vi "输出调用02.vi"(0 "输出簇":cluster{"用户名":string, "项目名称":string}, 7 "数组":string[][](array[string]), 9 "字符串":string, 11 "输出簇 2":T1, 12 "Str引用句柄":refnum<vi>) -> ()   [LabVIEW 2020]
uses:
  <vilib>/Utility/miscctls.llb/LVDateTimeRec.ctl
  <vilib>/numeric/Random Number (Range) DBL.vi
panel:
  out "压力":dbl
  out "数组 6":dbl[][](array[numeric])
  out "水质":dbl
  out "温度":dbl
  out "输出 3":dbl
  out "输出 2":dbl
  out "创建的路径":path
  out "路径 2":path
  out "路径":path
  out "错误输出":errorcluster
  out "数组 5":dbl[](array[numeric])
  out "数组 4":dbl[](array[numeric])
  out "文本":string[](array[string])
  out "数组 3":dbl[](array[numeric])
  out "数组 2":dbl[](array[numeric])
  out "错误输出 2":errorcluster caption="错误输出"
  out "元素":string
  out "数值 3":i32
  out "Numeric":i32
  in  "数值":u32
  out "输出 1":dbl
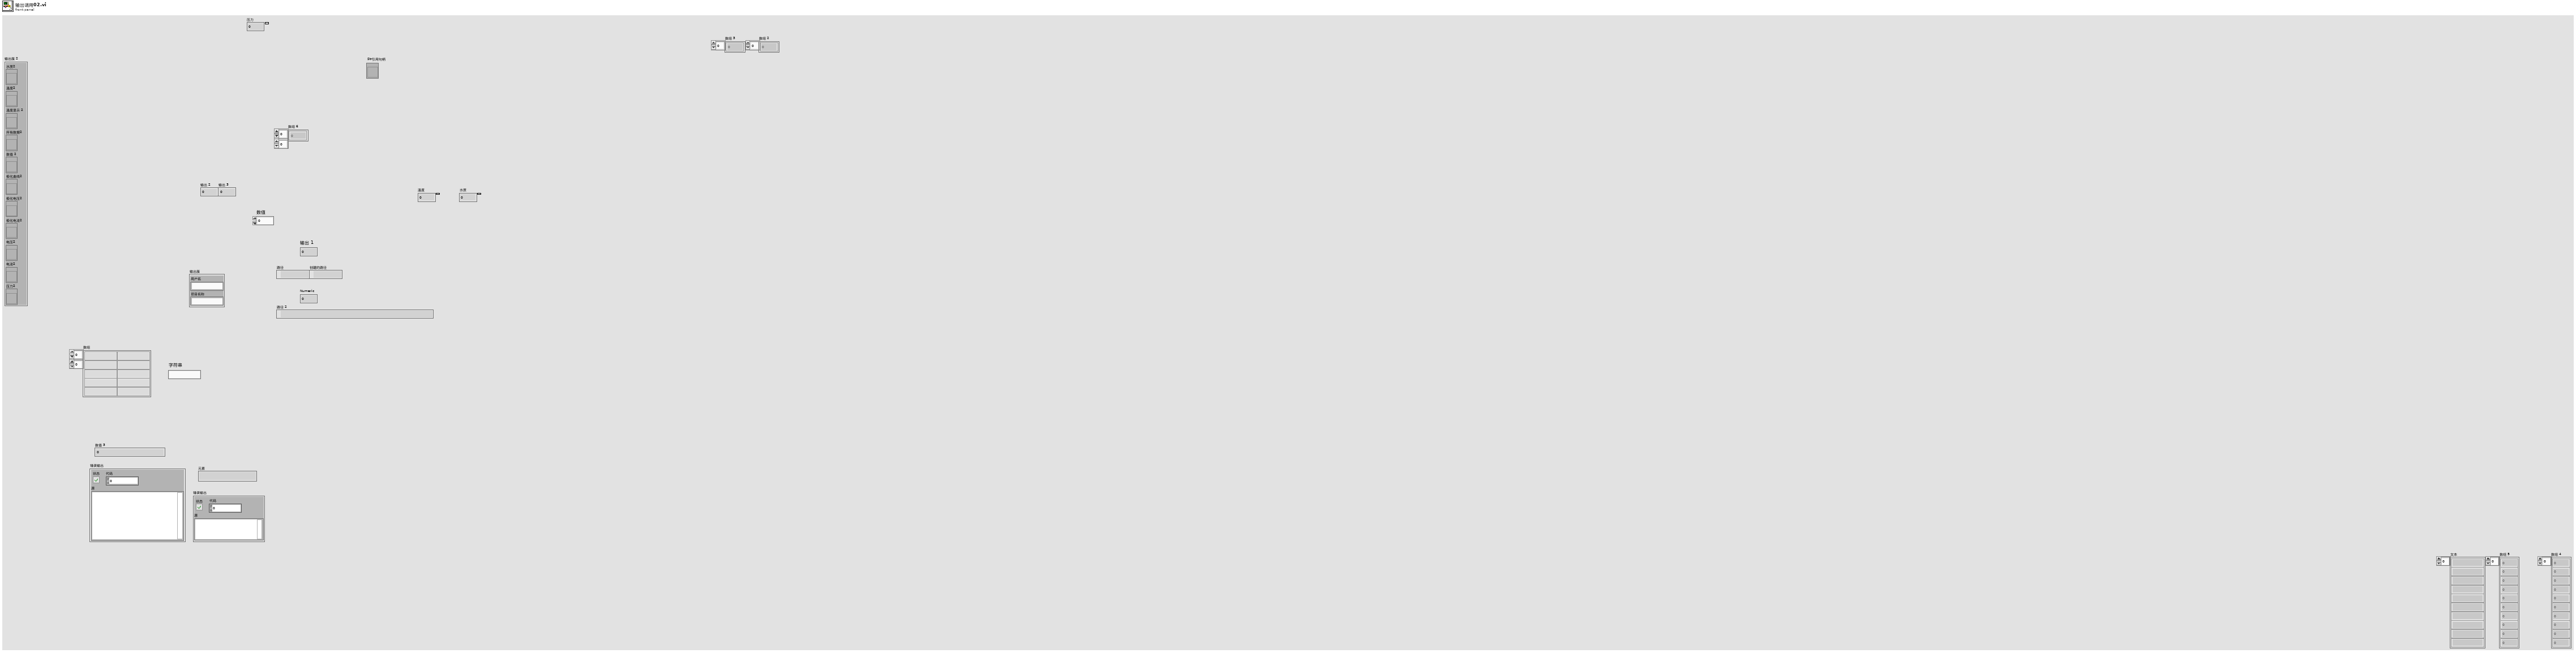
[diagram p1: front panel]
types:
  T1 = cluster{"水质2":refnum<vi>, "温度2":refnum<vi>, "温度显示 2":refnum<vi>, "所有数据2":refnum<vi>, "数值 2":refnum<vi>, "极化曲线2":refnum<vi>, "极化电压2":refnum<vi>, "极化电流2":refnum<vi>, "电压2":refnum<vi>, "电流2":refnum<vi>, "压力2":refnum<vi>}
  T2 = enum16{"open", "replace", "create", "open or create", "replace or create", "replace or create with confirmation"}
  T3 = typedef "LVDateTimeRec.ctl" = cluster{"fractional second":dbl, "second":i32, "minute":i32, "hour":i32, "day of month":i32, "month":i32, "year":i32, "day of week":i32, "day of year":i32, "DST":i32}
  T4 = enum16{"open", "open or create", "create or replace", "create", "open (read-only)"}
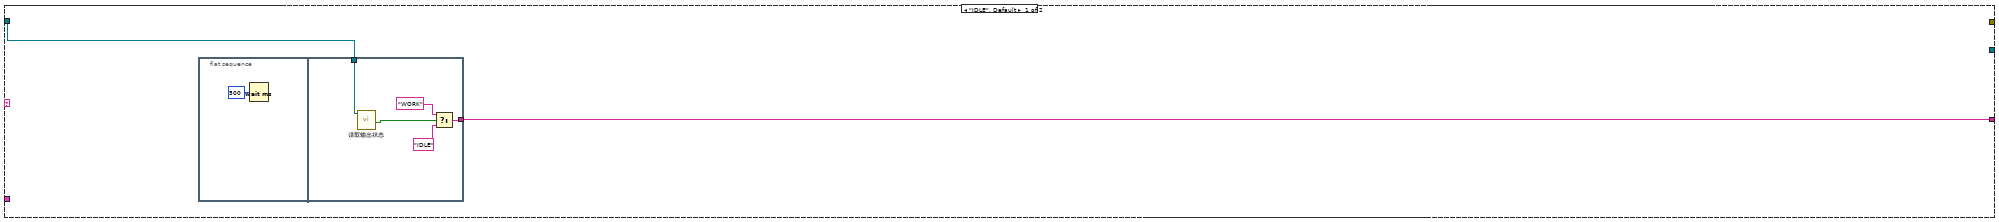
[diagram p2: hidden frame]
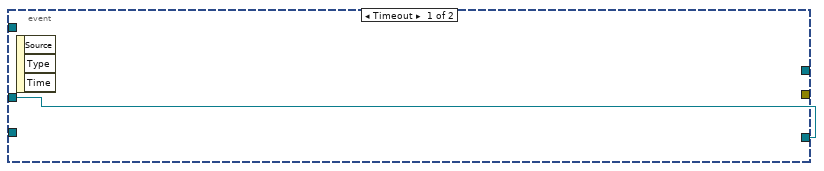
[diagram p3: hidden frame]
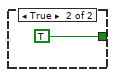
[diagram p5: hidden frame]
diagram:
  w17 = "\\" ("string")
  (unwired) dbl[] [] ("数组 4")
  n1 = Unbundle By Name("输出簇") -> ("用户名"=w14:string, "项目名称"=w13:string)
  n2 = Get Date/Time In Seconds() -> (seconds since 1Jan1904=w35:timestamp)
  n3 = Format Date/Time String(time format string (%c)="%y-%m-%d[%H-%M]", seconds (now)=w35) -> (date/time string=w16:string)  [unwired: 1 in]
  n4 = Concatenate Strings("C:\\Users\\526computer\\Desktop", w17, "TEMPDATA\\" ("string"), w14, w17, w13, w17, "CH2\\" ("string"), w16) -> (w33:string)
  n5 = String To Path(string=w33) -> (path=w32:path)
  n6 = Create Folder(path (use dialog)=w32) -> (created path=w4:path)  [unwired: 2 in, 2 out]
  "创建的路径" <- w4
  n7 = Path To String(path=w4) -> (string=w31:string)
  n8 = Concatenate Strings(w31, "\\" ("string"), "索引02.txt" ("string")) -> (w23:string)
  n9 = Path To String(path=w4) -> (string=w2:string)
  n10 = String To Path(string=w23) -> (path=w22:path)
  "路径 2" <- w22
  n11 = property on="输出簇 2" class="Clust (严格)"() -> ("Value"=w6:T1)  [unwired: 2 in, 2 out]
  n12 = property class="Str"(reference="Str引用句柄", "Value"=w2) -> ()  [unwired: 1 in, 2 out]
  n13 = Unbundle By Name(w6) -> ("极化曲线2"=w12:refnum<vi>)
  n14 = property on="数组 6" class="Arr (严格)"("Value"=dbl[][] [] ("数组 6")) -> (error out=w8:errorcluster)  [unwired: 2 in, 1 out]
  n15 = Open/Create/Replace File(file path (use dialog)=w22, operation (0:open)=T2."replace or create") -> (refnum out=w21:refnum<file>)  [unwired: 4 in, 2 out]
  n16 = while {
    tunnel: w45 -> [w66]
    tunnel: w21 -> [w65]
    tunnel: [w64] -> w19
    tunnel: [w63] -> w20
    shift-right: [w61] -> _
    shift-left: w12 -> [w62]
    tunnel: w8 -> [_]
    stop <- FALSE stop-if-true
    n17 = event shown="[1] \"数值\": 值改变" {
      selector: _ -> [_ _]
      dyn-events: _ -> [_ _]
      timeout: 100 -> [_ _]
      tunnel: w66 -> [_ _]
      tunnel: w65 -> [_ w84]
      tunnel: [_ w78] -> w64
      tunnel: [_ w77] -> w63
      tunnel: w62 -> [w69 w73]
      tunnel: [w69 w72] -> w61
      event Timeout {
        n18 = event-data() -> ()  [unwired: 1 in, 3 out]
      }
      event "数值": Value Change {
        n19 = event-data() -> ()  [unwired: 1 in, 6 out]
        n20 = local read "输出 3"() -> (w74:dbl)
        n21 = local read "输出 2"() -> (w75:dbl)
        n22 = property on="Numeric" class="DigNum (严格)"() -> ("Value"=w83:i32)  [unwired: 2 in, 2 out]
        n23 = Build Array(w75, w74) -> (w76:dbl[])
        n24 = Format Into String(w83) -> (resulting string=w82:string)  [unwired: 3 in, 1 out]
        n25 = property on="数组 6" class="Arr (严格)"() -> ("Value"=w71:dbl[][])  [unwired: 2 in, 2 out]
        n26 = Write to Text File(file (use dialog)=w84, text=w82) -> (refnum out=w81:refnum<file>, error out=w80:errorcluster)  [unwired: 2 in, 1 out]
        n27 = Insert Into Array(array=w71, new element=w76) -> (w70:dbl[][])  [unwired: 2 in]
        n28 = property on="数组 6" class="Arr (严格)"("Value"=w70) -> ()  [unwired: 2 in, 2 out]
        n29 = Write to Text File(file (use dialog)=w81, text="\r\n", error in=w80) -> (refnum out=w78:refnum<file>, error out=w77:errorcluster)  [unwired: 1 in, 1 out]
        n30 = property class="Arr (严格)"(reference=w73, "Value"=w70) -> (reference out=w72:refnum<vi>)  [unwired: 1 in, 1 out]
      }
    }
  }
  n31 = Path To String(path=w4) -> (string=w26:string)
  n32 = Concatenate Strings(w26, "\\" ("string"), "数据02.txt" ("string")) -> (w25:string)
  n33 = String To Path(string=w25) -> (path=w24:path)
  "路径" <- w24
  n34 = Close File(refnum=w19, error in=w20) -> ()  [unwired: 2 out]
  n35 = Open/Create/Replace File(file path (use dialog)=w24, operation (0:open)=T2."replace or create" ("操作(0:open)")) -> (refnum out=w10:refnum<file>, error out=w40:errorcluster)  [unwired: 4 in, 1 out]
  n36 = flat-sequence {
    tunnel: [w89] -> w60
    tunnel: [w86] -> w57
    tunnel: w60 -> [w93]
    tunnel: [w93] -> w59
    tunnel: [w92] -> w58
    tunnel: w57 -> [w92]
    tunnel: ["字符串"] -> w43
    tunnel: w59 -> [w95]
    tunnel: w58 -> [w96]
    tunnel: [w96] -> w56
    tunnel: [w95] -> w55
    tunnel: [w94] -> w44
    tunnel: w43 -> [w94]
    tunnel: w56 -> [w103]
    tunnel: w55 -> [w104]
    tunnel: [w106] -> w54
    tunnel: [w105] -> w53
    tunnel: [w104] -> w51
    tunnel: [w103] -> w49
    tunnel: [w102] -> w45
    tunnel: w44 -> [w101]
    tunnel: w54 -> [w119]
    tunnel: w53 -> [w118]
    tunnel: [w115] -> w52
    tunnel: w51 -> [w115]
    tunnel: [w114] -> w50
    tunnel: w49 -> [w114]
    tunnel: [w109] -> w48
    tunnel: [w108] -> w47
    tunnel: ["输出簇 2"] -> w11
    tunnel: w52 -> [w148]
    tunnel: w50 -> [w152]
    tunnel: w48 -> [w151]
    tunnel: w47 -> [w150]
    tunnel: [w149] -> w46
    tunnel: [w145] -> w37
    tunnel: w11 -> [w144]
    tunnel: w46 -> [w205]
    tunnel: w37 -> [w203]
    frame #0 {
      n37 = property on="数值" class="DigNum (严格)"("Value"=i64 0 ("数值")) -> ()  [unwired: 2 in, 2 out]
      n38 = Index Array(array="数组", index (col)=5 ("禁用的索引 (列)")) -> (element=w86:string[])  [unwired: 1 in]
      n39 = Index Array(array="数组", index (col)=3 ("禁用的索引 (列)")) -> (element=w89:string[])  [unwired: 1 in]
    }
    frame #1 {
      n40 = VISA Close(VISA resource name="字符串") -> ()  [unwired: 1 in, 1 out]
    }
    frame #2 {
    }
    frame #3 {
      n41 = VISA Open(VISA resource name=w101) -> (VISA resource name=w102:refnum<visa-resource-name>, error out=w99:errorcluster)  [unwired: 4 in]
      n42 = call "remote.vi"("error in (no error)"=w99, "VISA resource name"=w102) -> ("error out"=w97:errorcluster, "VISA resource name out"=w98:refnum<visa-resource-name>)  [unwired: 8 in]
      n43 = call "enableoutput.vi"("error in (no error)"=w97, "Enable OutPut(True)"=FALSE, "VISA resource name"=w98) -> ("error out"=w105:errorcluster, "VISA resource name out"=w106:refnum<visa-resource-name>)  [unwired: 7 in]
    }
    frame #4 {
      n44 = flat-sequence {
        tunnel: w119 -> [w124]
        tunnel: w118 -> [w123]
        tunnel: [w121] -> w117
        tunnel: [w120] -> w116
        tunnel: w117 -> [w130]
        tunnel: w116 -> [w129]
        tunnel: [w126] -> w113
        tunnel: [w125] -> w112
        tunnel: w113 -> [w136]
        tunnel: w112 -> [w135]
        tunnel: [w133] -> w111
        tunnel: [w132] -> w110
        tunnel: w111 -> [w142]
        tunnel: w110 -> [w141]
        tunnel: [w138] -> w109
        tunnel: [w137] -> w108
        frame #0 {
          n45 = call "priority.vi"("error in (no error)"=w123, "字符串"="CURR", "VISA resource name"=w124) -> ("error out"=w120:errorcluster, "VISA resource name out"=w121:refnum<visa-resource-name>)  [unwired: 7 in]
        }
        frame #1 {
          n46 = call "初始化电压电流.vi"("error in (no error)"=w129, "输入 2"=0.1, "输入 1"=15.0, "VISA resource name"=w130) -> ("error out"=w125:errorcluster, "VISA resource name out"=w126:refnum<visa-resource-name>)  [unwired: 6 in]
        }
        frame #2 {
          n47 = call "限制电流.vi"("error in (no error)"=w135, "OCP Delay(0)"=3.0, "数值"=120.0 ("OCP Level(0)"), "VISA resource name"=w136) -> ("error out"=w132:errorcluster, "VISA resource name out"=w133:refnum<visa-resource-name>)  [unwired: 6 in]
        }
        frame #3 {
          n48 = call "限制电压.vi"("error in (no error)"=w141, "OVP Delay(0)"=3.0, "OVP Level(0)"=20.0, "VISA resource name"=w142) -> ("error out"=w137:errorcluster, "VISA resource name out"=w138:refnum<visa-resource-name>)  [unwired: 6 in]
        }
      }
    }
    frame #5 {
      n49 = Unbundle By Name(w144) -> ("数值 2"=w143:refnum<vi>)
      n50 = Search 1D Array(1D array=w148, element=" " ("元素")) -> (index of element=w146:i32)  [unwired: 1 in]
      n51 = for {
        N: w146 -> [_]
        tunnel: w152 -> [w174] mode=indexing
        tunnel: w148 -> [w171] mode=indexing
        tunnel: w150 -> [w169]
        shift-right: [w164] -> w149
        shift-left: w151 -> [w170]
        tunnel: [w161] -> w145
        shift-right: [w155] -> _
        shift-left: w143 -> [w156]
        i -> [w154]
        n52 = Scan From String(input string=w174) -> (output 1=w173:dbl)  [unwired: 4 in, 3 out]
        n53 = Scan From String(input string=w171) -> (output 1=w168:dbl)  [unwired: 4 in, 3 out]
        "输出 1" <- w168
        n54 = Multiply(x=w173, y=1000.0) -> (x*y=w165:dbl)
        n55 = flat-sequence {
          tunnel: w170 -> [w179]
          tunnel: w169 -> [w178]
          tunnel: w168 -> [w177]
          tunnel: [w176] -> w167
          tunnel: [w175] -> w166
          tunnel: w167 -> [w182]
          tunnel: w166 -> [w183]
          tunnel: [w181] -> w163
          tunnel: [w180] -> w162
          tunnel: w165 -> [w193]
          tunnel: w163 -> [w192]
          tunnel: [w192] -> w160
          tunnel: [w191] -> w158
          tunnel: w162 -> [w191]
          tunnel: w160 -> [w198]
          tunnel: [w198] -> w159
          tunnel: w158 -> [w197]
          tunnel: [w197] -> w157
          tunnel: w156 -> [w196]
          tunnel: [w195] -> w155
          tunnel: w153 -> [w194]
          tunnel: [w201] -> w164
          tunnel: w159 -> [w202]
          tunnel: w157 -> [w200]
          tunnel: [w199] -> w161
          frame #0 {
            n56 = call "设置电流.vi"("error in (no error)"=w178, "输入 1"=w177, "VISA resource name"=w179) -> ("error out"=w175:errorcluster, "VISA resource name out"=w176:refnum<visa-resource-name>)  [unwired: 7 in]
          }
          frame #1 {
            n57 = First Call?() -> (First Call?: T/F=w184:bool)
            n58 = case shown="真" w184 {
              tunnel: w182 -> [w185 w190]
              tunnel: w183 -> [_ w189]
              tunnel: [w185 w187] -> w181
              tunnel: [_ w186] -> w180
              frame False {
              }
              frame True {
                n59 = call "enableoutput.vi"("error in (no error)"=w189, "Enable OutPut(True)"=TRUE, "VISA resource name"=w190) -> ("error out"=w186:errorcluster, "VISA resource name out"=w187:refnum<visa-resource-name>)  [unwired: 7 in]
              }
            }
          }
          frame #2 {
            n60 = Wait (ms)(milliseconds to wait=w193) -> ()  [unwired: 1 out]
          }
          frame #3 {
            n61 = property on="数值" class="DigNum (严格)"("Val(Sgnl)"=w194) -> ()  [unwired: 2 in, 2 out]
            n62 = property class="DigNum (严格)"(reference=w196, "Val(Sgnl)"=w194) -> (reference out=w195:refnum<vi>)  [unwired: 1 in, 1 out]
          }
          frame #4 {
            n63 = call "remote.vi"("error in (no error)"=w200, "VISA resource name"=w202) -> ("error out"=w199:errorcluster, "VISA resource name out"=w201:refnum<visa-resource-name>)  [unwired: 8 in]
          }
        }
        n64 = Increment(x=w154) -> (x+1=w153:i32)
      }
    }
    frame #6 {
      n65 = flat-sequence {
        tunnel: w205 -> [w209]
        tunnel: [w208] -> w204
        tunnel: w203 -> [w206]
        tunnel: w204 -> [w210]
        frame #0 {
          n66 = call "enableoutput.vi"("error in (no error)"=w206, "Enable OutPut(True)"=FALSE, "VISA resource name"=w209) -> ("VISA resource name out"=w208:refnum<visa-resource-name>)  [unwired: 7 in, 1 out]
        }
        frame #1 {
          n67 = VISA Close(VISA resource name=w210) -> ()  [unwired: 1 in, 1 out]
        }
        frame #2 {
          n68 = flat-sequence {
            tunnel: [w227] -> w221
            tunnel: [w226] -> w220
            tunnel: [w225] -> w219
            tunnel: [w224] -> w218
            tunnel: [w223] -> w217
            tunnel: w221 -> [w270]
            tunnel: w220 -> [w269]
            tunnel: [w287] -> w211
            tunnel: [w286] -> w212
            tunnel: w219 -> [w282]
            tunnel: [w281] -> w213
            tunnel: w218 -> [w273]
            tunnel: w217 -> [w274]
            tunnel: [w271] -> w214
            tunnel: [w272] -> w215
            tunnel: [w271] -> w216
            tunnel: w216 -> [w328]
            tunnel: w215 -> [w327]
            tunnel: w214 -> [w349]
            tunnel: w213 -> [w355]
            tunnel: w212 -> [w363]
            tunnel: w211 -> [w362]
            frame #0 {
              n69 = property on="路径" class="Path"() -> ("Value"=w222:path)  [unwired: 2 in, 2 out]
              n70 = Open/Create/Replace File(file path (use dialog)=w222, operation (0:open)=T2."open" ("操作(0:open)")) -> (refnum out=w230:refnum<file>, error out=w229:errorcluster)  [unwired: 4 in, 1 out]
              n71 = while {
                tunnel: w230 -> [w266]
                tunnel: w229 -> [w264]
                tunnel: [w263] -> w228
                tunnel: [w237] -> w227 mode=indexing
                tunnel: [w236] -> w226 mode=indexing
                tunnel: [w252] -> _
                tunnel: [w240] -> w225 mode=indexing
                tunnel: [w235] -> w224 mode=indexing
                tunnel: [w234] -> w223 mode=indexing
                i -> [w233]
                stop <- w253 stop-if-true
                n72 = Read from Text File(file (use dialog)=w266, count=1 ("计数"), error in=w264) -> (refnum out=w263:refnum<file>, text=w257:string[], error out=w252:errorcluster)  [unwired: 1 in, 1 out]
                n73 = Unbundle By Name(w252) -> ("status"=w260:bool, "code"=w262:i32)
                n74 = Equal?(x=w262, y=4) -> (x = y?=w259:bool)
                n75 = Index Array(array=w257, index=0 ("索引")) -> (element=w254:string)
                "元素" <- w254
                n76 = And(x=w260, y=w259) -> (x .and. y?=w258:bool)
                n77 = case shown="假" w258 {
                  tunnel: [FALSE TRUE] -> w253
                  frame False {
                  }
                  frame True {
                  }
                }
                n78 = Search/Split String(string=w254, search string/char (-)="电流：" ("正则表达式")) -> (substring before match=w249:string, match + rest of string=w239:string)  [unwired: 1 in, 1 out]
                n79 = Scan From String(format string="%d-%d-%d %d:%d:%d" ("格式字符串"), input string=w249) -> (error out=→"错误输出 2":errorcluster, output 1=w248:i32, output 2=w247:i32, output 3=w246:i32, output 4=w245:i32, output 5=w244:i32, output 6=w243:i32)  [unwired: 8 in, 2 out]
                n80 = Bundle By Name(cluster=T3 {"fractional second"=0.9035696983337402, "second"=34, "minute"=35, "hour"=15, "day of month"=21, "month"=2, "year"=2022, "day of week"=2, "day of year"=52, "DST"=0} ("日期时间记录"), "second"=w243, "minute"=w244, "hour"=w245, "day of month"=w246, "month"=w247, "year"=w248) -> (w241:T3)
                n81 = Scan From String(format string="电流：%f 电压：%f 温度：%f 水质：%f" ("格式字符串"), input string=w239) -> (error out=w232:errorcluster, output 1=w237:dbl, output 2=w236:dbl, output 3=w235:dbl, output 4=w234:dbl)  [unwired: 6 in, 2 out]
                n82 = call <vilib>:"Clear Errors.vi"("error in (no error)"=w232) -> ()  [unwired: 5 in, 2 out]
                n83 = Date/Time To Seconds(2:w241) -> (0:w240:timestamp)  [unwired: 1 in]
                "数值 3" <- w233
              }
              n84 = Close File(refnum=w228) -> ()  [unwired: 1 in, 2 out]
            }
            frame #1 {
              n85 = Array Size(array=w269) -> (size(s)=w289:i32)
              n86 = Array Size(array=w270) -> (size(s)=w292:i32)
              n87 = Array Size(array=w282) -> (size(s)=w284:i32)
              n88 = Decrement(x=w289) -> (x-1=w290:i32)
              n89 = Decrement(x=w292) -> (x-1=w291:i32)
              n90 = Decrement(x=w284) -> (x-1=w285:i32)
              n91 = Array Size(array=w273) -> (size(s)=w280:i32)
              n92 = Array Size(array=w274) -> (size(s)=w279:i32)
              n93 = Decrement(x=w280) -> (x-1=w278:i32)
              n94 = Decrement(x=w279) -> (x-1=w275:i32)
              n95 = Delete From Array(array=w273, length=1 ("长度"), index=w278) -> (array with subset deleted=w271:dbl[])  [unwired: 1 out]
              n96 = Delete From Array(array=w269, length=1 ("长度"), index=w290) -> (array with subset deleted=w286:dbl[])  [unwired: 1 out]
              n97 = Delete From Array(array=w270, length=1 ("长度"), index=w291) -> (array with subset deleted=w287:dbl[])  [unwired: 1 out]
              n98 = Delete From Array(array=w282, length=1 ("长度"), index=w285) -> (array with subset deleted=w281:timestamp[])  [unwired: 1 out]
              n99 = Delete From Array(array=w274, length=1 ("长度"), index=w275) -> (array with subset deleted=w272:dbl[])  [unwired: 1 out]
              "数组 3" <- w270
              "数组 2" <- w269
            }
            frame #2 {
              w314 = "极化" ("组名称输入（无标题）")
              w340 = "数据" ("组名称")
              n100 = property on="创建的路径" class="Path"() -> ("Value"=w294:path)  [unwired: 2 in, 2 out]
              n101 = Array Max & Min(array=w349) -> (max value=w321:dbl, max index (indices)=w319:i32, min value=w320:dbl, min index (indices)=w318:i32)
              n102 = Array Max & Min(array=w327) -> (max value=w325:dbl, max index (indices)=w323:i32, min value=w324:dbl, min index (indices)=w322:i32)
              n103 = Array Size(array=w355) -> (size(s)=w354:i32)
              n104 = Array Max & Min(array=w363) -> (max value=w376:dbl, max index (indices)=w371:i32, min value=w375:dbl, min index (indices)=w370:i32)
              n105 = Array Max & Min(array=w362) -> (max value=w378:dbl, max index (indices)=w372:i32, min value=w379:dbl, min index (indices)=w373:i32)
              n106 = Index Array(array=w355, index=0 ("索引")) -> (element=w352:timestamp)
              n107 = Build Array(w325, w324, w323, w322) -> (w336:dbl[])
              n108 = Build Array(w321, w320, w319, w318) -> (w337:dbl[])
              n109 = Decrement(x=w354) -> (x-1=w353:i32)
              n110 = Build Array(w375, w376, w371, w370) -> (w374:dbl[])
              n111 = Build Array(w379, w378, w373, w372) -> (w377:dbl[])
              n112 = Path To String(path=w294) -> (string=w295:string)
              n113 = Index Array(array=w355, index=w353) -> (element=w351:timestamp)
              n114 = Get Date/Time In Seconds() -> (seconds since 1Jan1904=w395:timestamp)
              n115 = Format Date/Time String(time format string (%c)="%Y-%m-%d-%H-%M-%S" ("时间格式字符串(%c)"), seconds (now)=w395) -> (date/time string=w297:string)  [unwired: 1 in]
              n116 = Concatenate Strings(w295, "\\" ("字符串"), w297, ".tdms" ("字符串")) -> (w396:string)
              n117 = String To Path(string=w396) -> (path=w397:path)
              n118 = Build Array(w352, w351) -> (w350:timestamp[])
              n119 = TDMS Open(5:FALSE ("创建索引文件？(T)"), 10:T4."create or replace" ("操作(0:open)"), 11:w397) -> (0:w303:errorcluster, 3:w305:refnum<k34>)  [unwired: 4 in]
              n120 = Build Array("电解水实验" ("组名称"), "孙成，王彪" ("组名称"), w297, "极化曲线" ("组名称")) -> (w296:string[])
              n121 = TDMS Set Properties(5:w296, 7:string[] ["Title", "Author", "Date/Time", "type"] ("属性名称"), 8:w303, 11:w305) -> (0:w302:errorcluster, 3:w304:refnum<k34>)  [unwired: 2 in, 2 out]
              n122 = TDMS Set Properties(5:w350, 7:string[] ["最小值", "最大值"] ("属性名称"), 8:w302, 9:"测试时间" ("通道名称"), 10:w340, 11:w304) -> (0:w386:errorcluster, 3:w387:refnum<k34>)  [unwired: 2 out]
              n123 = TDMS Set Properties(5:w377, 7:string[] ["最小值", "最大值", "最小索引", "最大索引"] ("属性名称"), 8:w386, 9:"电流" ("通道名称"), 10:w340, 11:w387) -> (0:w380:errorcluster, 3:w383:refnum<k34>)  [unwired: 2 out]
              n124 = TDMS Set Properties(5:w374, 7:string[] ["最小值", "最大值", "最小索引", "最大索引"] ("属性名称"), 8:w380, 9:"电压" ("通道名称"), 10:w340, 11:w383) -> (0:w343:errorcluster, 3:w344:refnum<k34>)  [unwired: 2 out]
              n125 = TDMS Set Properties(5:w337, 7:string[] ["最小值", "最大值", "最小索引", "最大索引"] ("属性名称"), 8:w343, 9:"温度" ("通道名称"), 10:w340, 11:w344) -> (0:w341:errorcluster, 3:w342:refnum<k34>)  [unwired: 2 out]
              n126 = TDMS Set Properties(5:w336, 7:string[] ["最小值", "最大值", "最小索引", "最大索引"] ("属性名称"), 8:w341, 9:"水质" ("通道名称"), 10:w340, 11:w342) -> (0:w338:errorcluster, 3:w339:refnum<k34>)  [unwired: 2 out]
              n127 = TDMS Write(0:w339, 5:"数据" ("组名称输入（无标题）"), 7:string[] ["电流"] ("通道名输入（无标题）"), 9:w362, 11:w338) -> (4:w366:refnum<k34>, 15:w365:errorcluster)  [unwired: 1 in, 2 out]
              n128 = TDMS Write(0:w366, 5:"数据" ("组名称输入（无标题）"), 7:string[] ["电压"] ("通道名输入（无标题）"), 9:w363, 11:w365) -> (4:w358:refnum<k34>, 15:w357:errorcluster)  [unwired: 1 in, 2 out]
              n129 = TDMS Write(0:w358, 5:"数据" ("组名称输入（无标题）"), 7:string[] ["测试时间"] ("通道名输入（无标题）"), 9:w355, 11:w357) -> (4:w330:refnum<k34>, 15:w329:errorcluster)  [unwired: 1 in, 2 out]
              n130 = TDMS Write(0:w330, 5:"数据" ("组名称输入（无标题）"), 7:string[] ["温度"] ("通道名输入（无标题）"), 9:w328, 11:w329) -> (4:w326:refnum<k34>, 15:w335:errorcluster)  [unwired: 1 in, 2 out]
              n131 = TDMS Write(0:w326, 5:"数据" ("组名称输入（无标题）"), 7:string[] ["水质"] ("通道名输入（无标题）"), 9:w327, 11:w335) -> (4:w311:refnum<k34>, 15:w310:errorcluster)  [unwired: 1 in, 2 out]
              n132 = flat-sequence {
                tunnel: [w399] -> w317
                tunnel: w317 -> [w406]
                tunnel: [w405] -> w307
                tunnel: [w404] -> w306
                frame #0 {
                  n133 = property on="路径 2" class="Path"() -> ("Value"=w398:path)  [unwired: 2 in, 2 out]
                  n134 = Open/Create/Replace File(file path (use dialog)=w398, operation (0:open)=T2."open" ("操作(0:open)")) -> (refnum out=w403:refnum<file>)  [unwired: 4 in, 2 out]
                  n135 = Read from Text File(file (use dialog)=w403, count=-1 ("计数")) -> (refnum out=w400:refnum<file>, text=w399:string[])  [unwired: 2 in, 2 out]
                  "文本" <- w399
                  n136 = Close File(refnum=w400) -> ()  [unwired: 1 in, 2 out]
                }
                frame #1 {
                  n137 = for {
                    tunnel: w406 -> [w415] mode=indexing
                    tunnel: [w413] -> w405 mode=indexing
                    tunnel: [w412] -> w404 mode=indexing
                    n138 = Scan From String(format string="%d" ("格式字符串"), input string=w415) -> (output 1=w411:i32)  [unwired: 3 in, 3 out]
                    n139 = property on="数组 3" class="Arr (严格)"() -> ("Value"=w407:dbl[])  [unwired: 2 in, 2 out]
                    n140 = Decrement(x=w411) -> (x-1=w410:i32)
                    n141 = Decrement(x=w411) -> (x-1=w409:i32)
                    n142 = Index Array(array=w407, index=w410) -> (element=w413:dbl)
                    n143 = property on="数组 2" class="Arr (严格)"() -> ("Value"=w408:dbl[])  [unwired: 2 in, 2 out]
                    n144 = Index Array(array=w408, index=w409) -> (element=w412:dbl)
                  }
                  "数组 5" <- w405
                  "数组 4" <- w404
                }
              }
              n145 = TDMS Write(0:w311, 5:w314, 7:string[] ["电流"] ("通道名输入（无标题）"), 9:w307, 11:w310) -> (4:w316:refnum<k34>, 15:w315:errorcluster)  [unwired: 1 in, 2 out]
              n146 = TDMS Write(0:w316, 5:w314, 7:string[] ["电压"] ("通道名输入（无标题）"), 9:w306, 11:w315) -> (4:w309:refnum<k34>, 15:w308:errorcluster)  [unwired: 1 in, 2 out]
              n147 = TDMS Close(8:w308, 11:w309) -> (0:→"错误输出":errorcluster)  [unwired: 1 out]
            }
          }
        }
        frame #3 {
          n148 = Request Deallocation(TRUE ("标志")) -> ()
        }
        frame #4 {
          n149 = Stop(stop? (T)=TRUE ("停止？(T)")) -> ()
        }
      }
    }
  }
  n150 = property on="输出簇 2" class="Clust (严格)"() -> ("Value"=w7:T1)  [unwired: 2 in, 2 out]
  n151 = while {
    shift-right: [w421] -> _
    shift-left: "IDLE" -> [w427]
    tunnel: w45 -> [w426]
    tunnel: w10 -> [w425]
    tunnel: w40 -> [w424]
    tunnel: [w423] -> w39
    tunnel: [w422] -> w38
    tunnel: w7 -> [w418]
    i -> [w420]
    stop <- FALSE stop-if-true
    n152 = Wait (ms)(milliseconds to wait=u32 500 ("等待时间（毫秒）")) -> ()  [unwired: 1 out]
    n153 = case shown="\"WORK\"" w427 {
      tunnel: [w430 w483] -> w421
      tunnel: w426 -> [w429 w491]
      tunnel: w425 -> [_ w490]
      tunnel: w424 -> [_ w488]
      tunnel: [_ w485] -> w423
      tunnel: [_ w484] -> w422
      tunnel: w418 -> [_ w470]
      frame "IDLE", Default {
        n154 = flat-sequence {
          tunnel: [w433] -> w430
          tunnel: w429 -> [w432]
          frame #0 {
            n155 = Wait (ms)(milliseconds to wait=u32 500 ("等待时间（毫秒）")) -> ()  [unwired: 1 out]
          }
          frame #1 {
            n156 = call "读取输出状态.vi"("VISA resource name"=w432) -> ("x = y?"=w436:bool)  [unwired: 7 in, 3 out]
            n157 = Select(t="WORK", s=w436, f="IDLE") -> (s? t:f=w433:string)
          }
        }
      }
      frame "WORK" {
        n158 = Unbundle By Name(w470) -> ("所有数据2"=w448:refnum<vi>, "极化电压2"=w446:refnum<vi>, "极化电流2"=w469:refnum<vi>, "电压2"=w468:refnum<vi>, "电流2"=w467:refnum<vi>, "水质2"=w447:refnum<vi>, "温度2"=w445:refnum<vi>, "压力2"=w438:refnum<vi>)  [unwired: 3 out]
        n159 = flat-sequence {
          tunnel: [w503] -> w494
          tunnel: [w502] -> w493
          tunnel: w491 -> [w501]
          tunnel: w490 -> [w499]
          tunnel: [w500] -> w489
          tunnel: w488 -> [w500]
          tunnel: [w499] -> w487
          tunnel: [w495] -> w486
          tunnel: w469 -> [w498]
          tunnel: [w495] -> w463
          tunnel: [w495] -> w437
          tunnel: w494 -> [w515]
          tunnel: w493 -> [w514]
          tunnel: [w512] -> w482
          tunnel: [w511] -> w480
          tunnel: w489 -> [w509]
          tunnel: w487 -> [w510]
          tunnel: [w510] -> w478
          tunnel: [w509] -> w476
          tunnel: [w508] -> w474
          tunnel: w486 -> [w508]
          tunnel: [w505] -> w472
          tunnel: [w505] -> w466
          tunnel: [w507] -> w464
          tunnel: w463 -> [w507]
          tunnel: [w505] -> w461
          tunnel: w446 -> [w506]
          tunnel: w437 -> [w505]
          tunnel: w482 -> [w532]
          tunnel: [w532] -> w481
          tunnel: w480 -> [w531]
          tunnel: [w531] -> w479
          tunnel: w478 -> [w530]
          tunnel: [w530] -> w477
          tunnel: w476 -> [w529]
          tunnel: [w529] -> w475
          tunnel: w474 -> [w528]
          tunnel: [w528] -> w473
          tunnel: w472 -> [w527]
          tunnel: [w527] -> w471
          tunnel: w468 -> [w526]
          tunnel: w467 -> [w518]
          tunnel: w466 -> [w523]
          tunnel: [w517] -> w465
          tunnel: w464 -> [w517]
          tunnel: [w516] -> w462
          tunnel: w461 -> [w516]
          tunnel: [w620] -> w460
          tunnel: w481 -> [w620]
          tunnel: w479 -> [w603]
          tunnel: w477 -> [w607]
          tunnel: w475 -> [w606]
          tunnel: w473 -> [w605]
          tunnel: w471 -> [w593]
          tunnel: [w604] -> w458
          tunnel: [w603] -> w456
          tunnel: [w602] -> w484
          tunnel: [w589] -> w454
          tunnel: w465 -> [w589]
          tunnel: [w588] -> w452
          tunnel: w462 -> [w588]
          tunnel: [w581] -> w450
          tunnel: w447 -> [w580]
          tunnel: w445 -> [w561]
          tunnel: [w560] -> w443
          tunnel: [w559] -> w441
          tunnel: [w545] -> w439
          tunnel: w438 -> [w544]
          tunnel: w460 -> [w629]
          tunnel: [w629] -> w459
          tunnel: w458 -> [w628]
          tunnel: [w628] -> w457
          tunnel: w456 -> [w627]
          tunnel: [w627] -> w455
          tunnel: w454 -> [w626]
          tunnel: [w626] -> w453
          tunnel: w452 -> [w625]
          tunnel: [w625] -> w451
          tunnel: w450 -> [w624]
          tunnel: [w624] -> w449
          tunnel: [w623] -> w444
          tunnel: w443 -> [w623]
          tunnel: [w622] -> w442
          tunnel: w441 -> [w622]
          tunnel: [w621] -> w440
          tunnel: w439 -> [w621]
          tunnel: [w651] -> w492
          tunnel: w459 -> [w651]
          tunnel: w457 -> [w650]
          tunnel: w455 -> [w649]
          tunnel: [w648] -> w485
          tunnel: w453 -> [w643]
          tunnel: w451 -> [w640]
          tunnel: w449 -> [w634]
          tunnel: w448 -> [w633]
          tunnel: w444 -> [w632]
          tunnel: w442 -> [w631]
          tunnel: w440 -> [w630]
          tunnel: w492 -> [w656]
          tunnel: [w652] -> w483
          frame #0 {
            w504 = 0 items=["Current", "Power", "Voltage", "Capacity", "Temperature", "Time"] ("Fetch Type")
            n160 = call-poly <vilib>:"Random Number (Range).vi"("lower bound (0)"=10.0, "upper bound (100)"=20.0) -> ("number"=w495:dbl)  [unwired: 9 in]
            "输出 2" <- w495
            n161 = call "fetch.vi"("Fetch Type"=w504, "VISA resource name"=w501) -> ("error out"=w502:errorcluster, "VISA resource name out"=w503:refnum<visa-resource-name>)  [unwired: 7 in, 1 out]
            n162 = property class="DigNum (严格)"(reference=w498, "Value"=w495) -> ()  [unwired: 1 in, 2 out]
          }
          frame #1 {
            w513 = 2 items=["Current", "Power", "Voltage", "Capacity", "Temperature", "Time"] ("Fetch Type")
            n163 = property class="DigNum (严格)"(reference=w506, "Value"=w505) -> ()  [unwired: 1 in, 2 out]
            n164 = call "fetch.vi"("error in (no error)"=w514, "Fetch Type"=w513, "VISA resource name"=w515) -> ("error out"=w511:errorcluster, "VISA resource name out"=w512:refnum<visa-resource-name>)  [unwired: 6 in, 1 out]
            "输出 3" <- w505
          }
          frame #2 {
            n165 = property class="Arr (严格)"(reference=w526) -> (reference out=w525:refnum<vi>, "Value"=w524:dbl[])  [unwired: 1 in, 1 out]
            n166 = Insert Into Array(array=w524, new element=w523) -> (w522:dbl[])  [unwired: 1 in]
            n167 = property class="Arr (严格)"(reference=w518) -> (reference out=w519:refnum<vi>, "Value"=w520:dbl[])  [unwired: 1 in, 1 out]
            n168 = property class="Arr (严格)"(reference=w525, "Value"=w522) -> ()  [unwired: 1 in, 2 out]
            n169 = Insert Into Array(array=w520, new element=w517) -> (w521:dbl[])  [unwired: 1 in]
            n170 = property class="Arr (严格)"(reference=w519, "Value"=w521) -> ()  [unwired: 1 in, 2 out]
          }
          frame #3 {
            (unwired) "时间：" ("字符串")
            n171 = Get Date/Time String() -> (date string=w567:string, time string=w565:string)  [unwired: 3 in]
            n172 = Get Date/Time String() -> (date string=w585:string, time string=w587:string)  [unwired: 3 in]
            n173 = call <vilib>:"Space Constant.vi"() -> ("String"=w579:string)
            n174 = Get Date/Time In Seconds() -> (seconds since 1Jan1904=w619:timestamp)
            n175 = Format Into String(w605) -> (resulting string=w616:string)  [unwired: 3 in, 1 out]
            n176 = Get Date/Time String() -> (date string=w550:string, time string=w552:string)  [unwired: 3 in]
            n177 = Concatenate Strings(w567, "  " ("字符串"), w565) -> (w571:string)
            n178 = Concatenate Strings(w579, "电流：" ("字符串"), w616) -> (w615:string)
            n179 = Concatenate Strings(w585, "  " ("字符串"), w587) -> (w581:string)
            n180 = call-poly <vilib>:"Random Number (Range).vi"("lower bound (0)"=20.0, "upper bound (100)"=30.0) -> ("number"=w535:dbl)  [unwired: 9 in]
            n181 = Format Into String(format string="%.2f" ("格式字符串"), w535) -> (resulting string=w559:string)  [unwired: 2 in, 1 out]
            n182 = Format Into String(format string="%.2f" ("格式字符串"), w535) -> (resulting string=w560:string)  [unwired: 2 in, 1 out]
            n183 = Concatenate Strings(w550, "  " ("字符串"), w552) -> (w546:string)
            n184 = Format Into String(format string="%.2f" ("格式字符串"), w535) -> (resulting string=w545:string)  [unwired: 2 in, 1 out]
            n185 = Format Date/Time String(time format string (%c)="%Y-%m-%d %H:%M:%S" ("时间格式字符串(%c)"), seconds (now)=w619) -> (date/time string=w617:string)  [unwired: 1 in]
            n186 = Write to Text File(file (use dialog)=w607, text=w617, error in=w606) -> (refnum out=w614:refnum<file>, error out=w613:errorcluster)  [unwired: 1 in, 1 out]
            n187 = Write to Text File(file (use dialog)=w614, text=w615, error in=w613) -> (refnum out=w610:refnum<file>, error out=w609:errorcluster)  [unwired: 1 in, 1 out]
            n188 = call <vilib>:"Space Constant.vi"() -> ("String"=w578:string)
            n189 = Format Into String(w593) -> (resulting string=w611:string)  [unwired: 3 in, 1 out]
            n190 = property on="温度" class="DigNum (严格)" props=["Value"]() -> ()  [unwired: 2 in, 3 out]
            n191 = Concatenate Strings(w559, "°C" ("字符串")) -> (w569:string)
            n192 = Concatenate Strings(w560, "MΩ*cm" ("字符串")) -> (w583:string)
            n193 = Concatenate Strings(w545, "bar" ("字符串")) -> (w548:string)
            n194 = property class="Arr (严格)"(reference=w561) -> (reference out=w562:refnum<vi>, "Value"=w564:string[][])  [unwired: 1 in, 1 out]
            n195 = property class="Arr (严格)"(reference=w580) -> (reference out=w592:refnum<vi>, "Value"=w590:string[][])  [unwired: 1 in, 1 out]
            n196 = Concatenate Strings(w578, "电压：" ("字符串"), w611) -> (w612:string)
            n197 = Write to Text File(file (use dialog)=w610, text=w612, error in=w609) -> (refnum out=w597:refnum<file>, error out=w596:errorcluster)  [unwired: 1 in, 1 out]
            n198 = property class="Arr (严格)"(reference=w544) -> (reference out=w555:refnum<vi>, "Value"=w553:string[][])  [unwired: 1 in, 1 out]
            n199 = Build Array(w571, w569) -> (w570:string[])
            n200 = Build Array(w581, w583) -> (w582:string[])
            n201 = Build Array(w546, w548) -> (w547:string[])
            n202 = call <vilib>:"Space Constant.vi"() -> ("String"=w577:string)
            n203 = Format Into String(w535) -> (resulting string=w601:string)  [unwired: 3 in, 1 out]
            n204 = property on="水质" class="DigNum (严格)" props=["Value"]() -> ()  [unwired: 2 in, 3 out]
            n205 = Insert Into Array(array=w564, new element=w570) -> (w563:string[][])  [unwired: 2 in]
            n206 = Insert Into Array(array=w590, new element=w582) -> (w591:string[][])  [unwired: 2 in]
            n207 = Insert Into Array(array=w553, new element=w547) -> (w554:string[][])  [unwired: 2 in]
            n208 = Concatenate Strings(w577, "温度：" ("字符串"), w601) -> (w600:string)
            n209 = Write to Text File(file (use dialog)=w597, text=w600, error in=w596) -> (refnum out=w595:refnum<file>, error out=w594:errorcluster)  [unwired: 1 in, 1 out]
            n210 = call <vilib>:"Space Constant.vi"() -> ("String"=w576:string)
            n211 = Format Into String(w535) -> (resulting string=w598:string)  [unwired: 3 in, 1 out]
            n212 = property class="Arr (严格)"(reference=w562, "Value"=w563) -> ()  [unwired: 1 in, 2 out]
            n213 = property on="压力" class="DigNum (严格)" props=["Value"]() -> ()  [unwired: 2 in, 3 out]
            n214 = property class="Arr (严格)"(reference=w592, "Value"=w591) -> ()  [unwired: 1 in, 2 out]
            n215 = property class="Arr (严格)"(reference=w555, "Value"=w554) -> ()  [unwired: 1 in, 2 out]
            n216 = Concatenate Strings(w576, "水质：" ("字符串"), w598) -> (w599:string)
            n217 = Write to Text File(file (use dialog)=w595, text=w599, error in=w594) -> (refnum out=w539:refnum<file>, error out=w538:errorcluster)  [unwired: 1 in, 1 out]
            n218 = call <vilib>:"Space Constant.vi"() -> ("String"=w542:string)
            n219 = Format Into String(w535) -> (resulting string=w541:string)  [unwired: 3 in, 1 out]
            n220 = Concatenate Strings(w542, "压力：" ("字符串"), w541) -> (w540:string)
            n221 = Write to Text File(file (use dialog)=w539, text=w540, error in=w538) -> (refnum out=w534:refnum<file>, error out=w533:errorcluster)  [unwired: 1 in, 1 out]
            n222 = Write to Text File(file (use dialog)=w534, text="\r\n", error in=w533) -> (refnum out=w602:refnum<file>, error out=w604:errorcluster)  [unwired: 1 in, 1 out]
          }
          frame #4 {
          }
          frame #5 {
            n223 = Multiply(x=w640, y=w643) -> (x*y=w637:dbl)
            n224 = Format Into String(format string="%.2f" ("格式字符串"), w643) -> (resulting string=w642:string)  [unwired: 2 in, 1 out]
            n225 = Merge Errors(w649, w650) -> (w648:errorcluster)
            n226 = Format Into String(format string="%.2f" ("格式字符串"), w640) -> (resulting string=w639:string)  [unwired: 2 in, 1 out]
            n227 = Format Into String(format string="%.2f" ("格式字符串"), w637) -> (resulting string=w636:string)  [unwired: 2 in, 1 out]
            n228 = property class="Arr (严格)"(reference=w633) -> (reference out=w646:refnum<vi>, "Value"=w647:string[][])  [unwired: 1 in, 1 out]
            n229 = Build Array(w634, w642, w639, w636, w631, w632, w630) -> (w635:string[])
            n230 = Insert Into Array(array=w647, new element=w635) -> (w645:string[][])  [unwired: 2 in]
            n231 = property class="Arr (严格)"(reference=w646, "Value"=w645) -> ()  [unwired: 1 in, 2 out]
          }
          frame #6 {
            n232 = call "读取输出状态.vi"("VISA resource name"=w656) -> ("x = y?"=w655:bool)  [unwired: 7 in, 3 out]
            n233 = Select(t="WORK", s=w655, f="IDLE") -> (s? t:f=w652:string)
          }
        }
      }
    }
    "Numeric" <- w420
  }
  n234 = Close File(refnum=w38, error in=w39) -> ()  [unwired: 2 out]
